vi "Inheritance test.vi"   [LabVIEW 2019, in "Instrument.OxfordVRM.lvclass"]
uses:
  Instrument.OxfordVRM.lvclass
  <userlib>/LevyLab/Instrument Framework/Instrument Types/Cryostat/Instrument.Cryostat.lvclass
  <userlib>/LevyLab/Instrument Framework/SMOs/Instrument/Instrument.lvclass
  <vilib>/JKI/JKI SMO/SMO/SMO.lvclass
  C:/Program Files (x86)/National Instruments/LabVIEW 2019/user.lib/LevyLab/Instrument Framework/Instrument Types/Cryostat/Instrument.Cryostat.lvclass
  C:/Program Files (x86)/National Instruments/LabVIEW 2019/user.lib/LevyLab/Instrument Framework/Instrument/Instrument.lvclass
  C:/Program Files (x86)/National Instruments/LabVIEW 2019/vi.lib/JKI/JKI SMO/SMO/SMO.lvclass
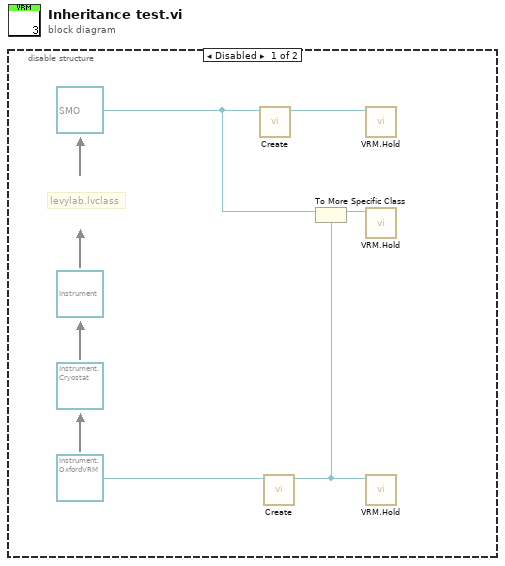
[diagram p0: block diagram]
diagram:
  n1 = disable-structure shown="Disabled" {
    frame Disabled {
      w4 = refnum<class "SMO.lvclass"> refnum ("SMO.lvclass")
      (unwired) refnum<class "Instrument.lvclass"> refnum ("Instrument.lvclass")
      (unwired) refnum<class "Instrument.Cryostat.lvclass"> refnum ("Instrument.Cryostat.lvclass")
      # "levylab.lvclass"
      n2 = call <vilib>:"Create.vi"("SMO"=w4) -> ("SMO out"=w5:refnum<class "SMO.lvclass">)  [unwired: 8 in, 2 out]
      n3 = call <vilib>:"Create.vi"("SMO"=refnum<class "Instrument.OxfordVRM.lvclass"> refnum ("Instrument.Oxford1820.lvclass")) -> ("SMO out"=w1:refnum<class "Instrument.OxfordVRM.lvclass">)  [unwired: 8 in, 2 out]
      n4 = To More Specific Class(target class=w1, reference=w4) -> (specific class reference=w2:refnum<class "Instrument.OxfordVRM.lvclass">)  [unwired: 1 in, 1 out]
      n5 = call "VRM.Hold.vi"("Instrument.VRM in"=w5) -> ()  [unwired: 8 in, 3 out]
      n6 = call "VRM.Hold.vi"("Instrument.VRM in"=w2) -> ()  [unwired: 8 in, 3 out]
      n7 = call "VRM.Hold.vi"("Instrument.VRM in"=w1) -> ()  [unwired: 8 in, 3 out]
    }
    frame Enabled {
    }
  }
